vi "Byte Buffer.Subset.Set.vi"(8 "error in (no error)":errorcluster, 9 "offset (0)":u64, 10 "string in":string, 11 "Byte Buffer in":refnum<class "Byte Buffer.lvclass">) -> (0 "error out":errorcluster, 1 "new buffer offset":u64, 2 "string out":string, 3 "Byte Buffer out":refnum<class "Byte Buffer.lvclass">)   [LabVIEW 2016, in "VeriStand Data.lvlib" / "Byte Buffer.lvclass"]
doc: "Writes the contents of the provided <B>string</B> to the <B>Byte Buffer</B> at the specified <B>offset</B>."
uses:
  Byte Buffer.lvclass
  Byte Buffer.lvclass/Byte Buffer.ctl
  Memory Management/Memory Management.Handle Return.vi
  VeriStand Data.lvlib
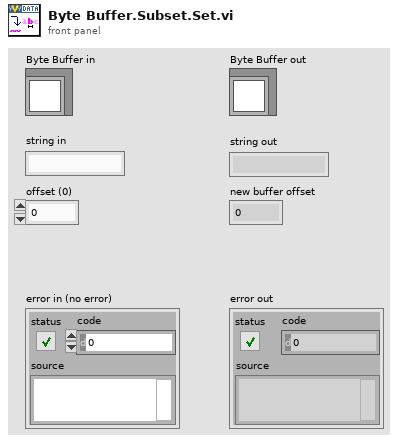
[diagram p1: front panel]
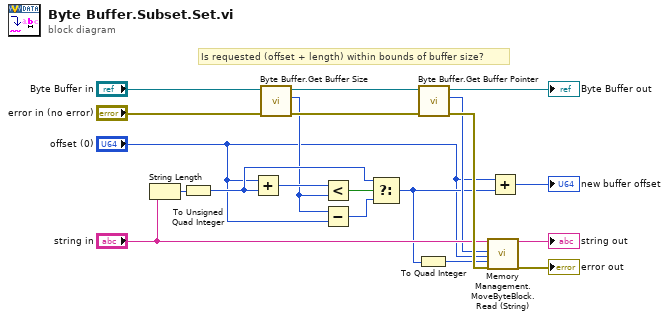
[diagram p0: block diagram]
diagram:
  # "Is requested (offset + length) within bounds of buffer size?"
  n1 = String Length(string="string in") -> (length=w13:i32)
  n2 = To Unsigned Quad Integer(1:w13) -> (0:w11:u64)
  n3 = Add(x="offset (0)", y=w11) -> (x+y=w12:u64)
  n4 = call "Byte Buffer.Get Buffer Size.vi"("error in (no error)"="error in (no error)", "Byte Buffer in"="Byte Buffer in") -> ("error out"=w6:errorcluster, "buffer size"=w5:u64, "Byte Buffer out"=w7:refnum<class "Byte Buffer.lvclass">)  [unwired: 7 in]
  n5 = Less?(x=w12, y=w5) -> (x < y?=w14:bool)
  n6 = Subtract(x=w5, y="offset (0)") -> (x-y=w10:u64)
  n7 = Select(t=w11, s=w14, f=w10) -> (s? t:f=w8:u64)
  n8 = To Quad Integer(1:w8) -> (0:w9:i64)
  n9 = call "Byte Buffer.Get Buffer Pointer.vi"("error in (no error)"=w6, "Byte Buffer in"=w7) -> ("error out"=w20:errorcluster, "buffer pointer"=w15:u64, "Byte Buffer out"=→"Byte Buffer out":refnum<class "Byte Buffer.lvclass">)  [unwired: 7 in]
  n10 = call "Memory Management.MoveByteBlock.Read (String).vi"("src in"="string in", "dst ptr in"=w15, "dst offset (0)"="offset (0)", "size"=w9, "error in (no error)"=w20) -> ("src out"=→"string out":string, "error out"=→"error out":errorcluster)  [unwired: 9 in, 4 out]
  n11 = Add(x="offset (0)", y=w8) -> (x+y=→"new buffer offset":u64)
